vi "GetQ_HP8722ET.vi"(0 "GPIB\nAddress":string="16") -> (1 "Frequency":dbl format="%.6e", 2 "Delta Frequency":dbl format="%.6e", 3 "Q factor":dbl=-6977319.0 format="%.6e")   [LabVIEW 2015]
panel:
  in  "# bytes\nto read":i32=200
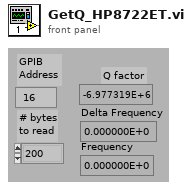
[diagram p1: front panel]
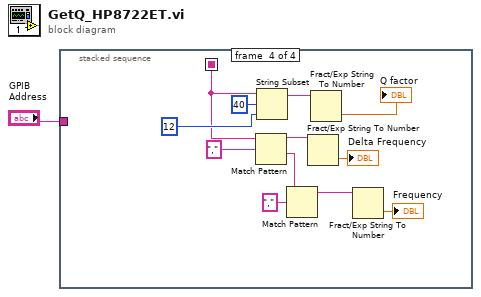
[diagram p0: block diagram]
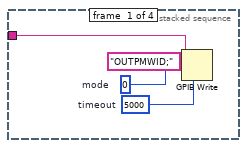
[diagram p2: hidden frame]
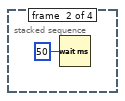
[diagram p3: hidden frame]
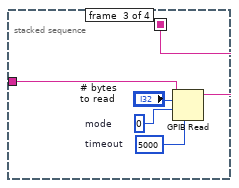
[diagram p4: hidden frame]
diagram:
  n1 = stacked-sequence {
    seq-local: [_ _ w7 _] -> [_ _ _ w19]
    tunnel: "GPIB\nAddress" -> [w5 _ w11 _]
    frame #0 {
      w3 = u32 5000  # timeout
      w4 = 0  # mode
      n2 = GPIB Write(0:w5, 1:"OUTPMWID;" ("data"), 2:w4, 4:w3) -> ()  [unwired: 1 in, 2 out]
    }
    frame #1 {
      n3 = Wait (ms)(milliseconds to wait=u32 50) -> ()  [unwired: 1 out]
    }
    frame #2 {
      w10 = 0  # mode
      w8 = u32 5000  # timeout
      n4 = GPIB Read(0:w11, 1:"# bytes\nto read", 2:w10, 4:w8) -> (5:w7:string)  [unwired: 1 in, 2 out]
    }
    frame #3 {
      n5 = Match Pattern(string=w19, regular expression=",") -> (before substring=w17:string, after substring=w14:string)  [unwired: 1 in, 2 out]
      n6 = String Subset(string=w19, offset (0)=40, length (rest)=12 ("length")) -> (substring=w21:string)
      n7 = Match Pattern(string=w14, regular expression=",") -> (before substring=w13:string)  [unwired: 1 in, 3 out]
      n8 = Fract/Exp String To Number(string=w17) -> (number=→"Delta Frequency":dbl)  [unwired: 3 in, 1 out]
      n9 = Fract/Exp String To Number(string=w21) -> (number=→"Q factor":dbl)  [unwired: 3 in, 1 out]
      n10 = Fract/Exp String To Number(string=w13) -> (number=→"Frequency":dbl)  [unwired: 3 in, 1 out]
    }
  }
